vi "DB_Create.vi"() -> ()   [LabVIEW 2020]
uses:
  <vilib>/addons/database/Auxilliary.llb/DB Tools Column Info.ctl
  <vilib>/addons/database/Auxilliary.llb/DB Tools DataTypes.ctl
  <vilib>/addons/database/Connection.llb/DB Tools Open Connec (String).vi
  <vilib>/addons/database/NI_Database_API.lvlib
panel:
  in  "column information":T1[](array[typedef])=[{"column name"="Nom", "data type"=enum."String", "size"=50, "allow null?"=FALSE}, {"column name"="Prénom", "data type"=enum."String", "size"=50, "allow null?"=FALSE}, {"column name"="age", "data type"=enum."Single (SGL)", "size"=0, "allow null?"=FALSE}, {"column name"="Sexe", "data type"=enum."String", "size"=1, "allow null?"=FALSE}, {"column name"="Métier", "data type"=enum."String", "size"=50, "allow null?"=FALSE}, {"column name"="Rémunération", "data type"=enum."Single (SGL)", "size"=0, "allow null?"=FALSE}]
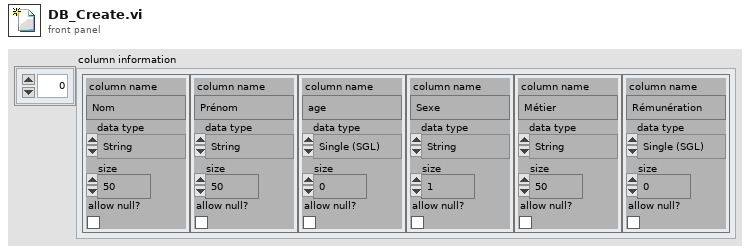
[diagram p1: front panel]
types:
  T1 = typedef "NI_Database_API.lvlib/DB Tools Column Info.ctl" = cluster{"column name":string, "data type":T2, "size":i32, "allow null?":bool}
  T2 = typedef "NI_Database_API.lvlib/DB Tools DataTypes.ctl" = enum16{"String", "Long (I32)", "Single (SGL)", "Double (DBL)", "Date/Time", "Binary"}
  T3 = typedef "NI_Database_API.lvlib/Conn ObjectReference.ctl" = refnum<k1>
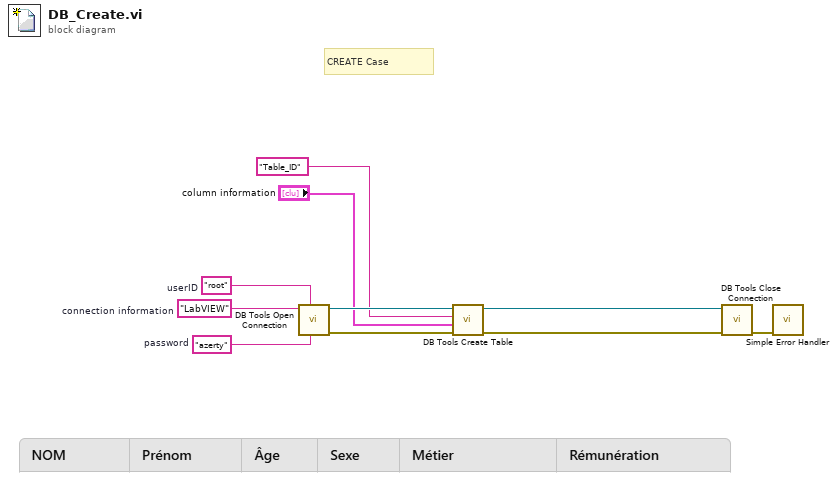
[diagram p0: block diagram]
diagram:
  w1 = "root"  # userID
  w3 = "azerty"  # password
  w2 = "LabVIEW"  # connection information
  # "CREATE Case"
  n1 = call-poly <vilib>:"DB Tools Open Connection.vi"("password"=w3, "userID"=w1, "connection information"=w2) -> ("error out"=w9:errorcluster, "connection reference"=w10:T3)  [unwired: 5 in]
  n2 = call <vilib>:"DB Tools Create Table.vi"("error in (no error)"=w9, "column information"="column information", "table"="Table_ID", "connection reference"=w10) -> ("error out"=w6:errorcluster, "connection reference out"=w8:T3)  [unwired: 4 in]
  n3 = call <vilib>:"DB Tools Close Connection.vi"("error in (no error)"=w6, "connection reference"=w8) -> ("error out"=w7:errorcluster)  [unwired: 5 in]
  n4 = call <vilib>:"Simple Error Handler.vi"("error in (no error)"=w7) -> ()  [unwired: 4 in, 5 out]
